vi "Describe Comparison.vi"(6 "Delta":variant, 7 "Style":enum16{"Diff", "Plain"}(ring), 9 "Actual":variant, 10 "Expected":variant) -> (2 "Description":string)   [LabVIEW 2020, in "Utilities.lvlib"]
uses:
  Utilities.lvlib
  <vilib>/Utility/Data Type/NI_Data Type.lvlib
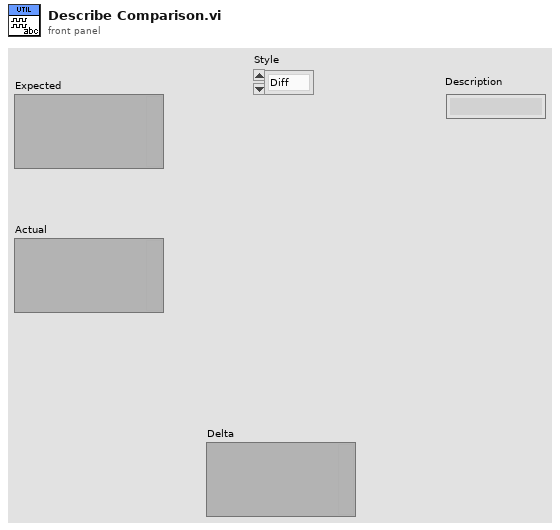
[diagram p1: front panel]
types:
  T1 = typedef "NI_Data Type.lvlib/Data Type.ctl" = enum8{"Invalid Type", "Void", "I8", "I16", "I32", "I64", "U8", "U16", "U32", "U64", "Single Float", "Double Float", "Extended Float", "Single Complex", "Double Complex", "Extended Complex", "Enum U8", "Enum U16", "Enum U32", "Enum U64", "Single Float With Unit", "Double Float With Unit", "Extended Float With Unit", "Single Complex with Unit", "Double Complex with Unit", "Extended Complex with Unit", "Boolean", "String", "Path", "Picture", "Tag", "Array", "Cluster", "Variant", "LV Variant", "Waveform", "Timestamp", "Digital Waveform", "Digital Data", "ExpressData", "Refnum", "External Data", "VI", "Poly VI", "LabVIEW Class Instance", "Fixed Point", "Set Collection", "Map Collection"}
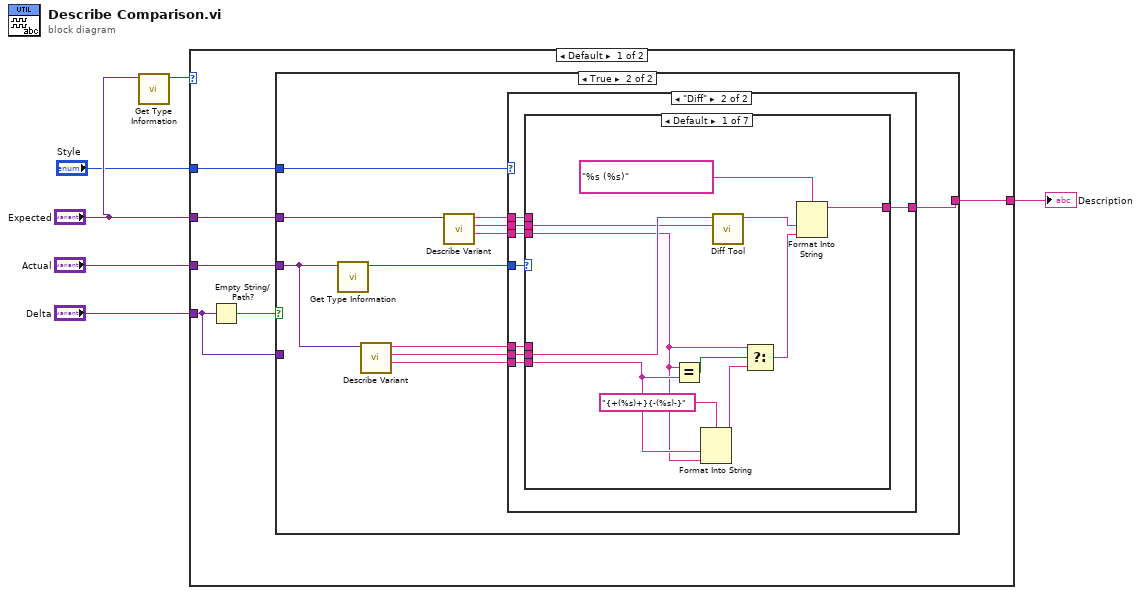
[diagram p0: block diagram]
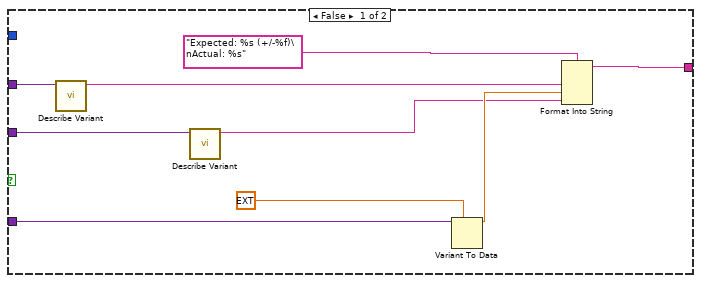
[diagram p2: hidden frame]
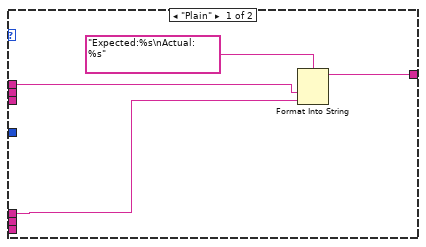
[diagram p3: hidden frame]
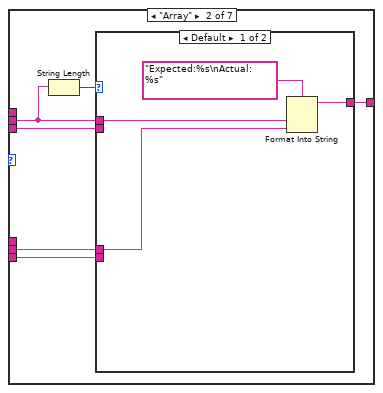
[diagram p4: hidden frame]
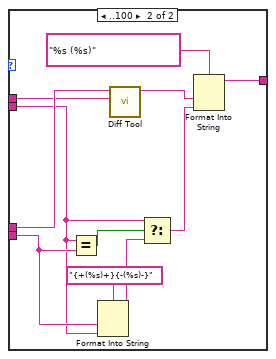
[diagram p5: hidden frame]
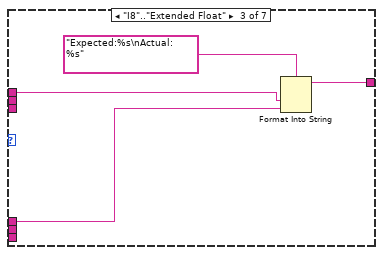
[diagram p6: hidden frame]
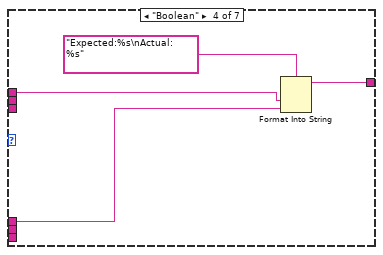
[diagram p7: hidden frame]
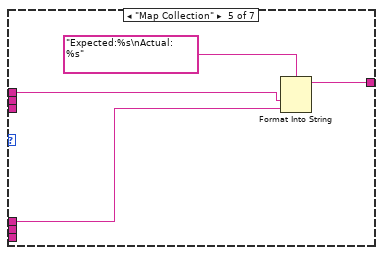
[diagram p8: hidden frame]
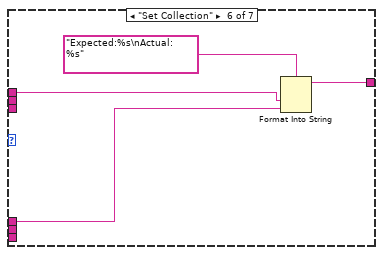
[diagram p9: hidden frame]
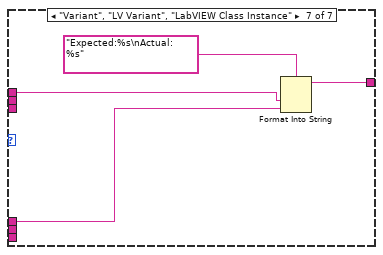
[diagram p10: hidden frame]
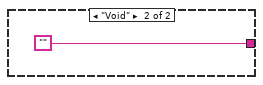
[diagram p11: hidden frame]
diagram:
  n1 = call <vilib>:"Get Type Information.vi"("variant"="Expected") -> ("type"=w2:T1)  [unwired: 6 in, 4 out]
  n2 = case shown="Default" w2 {
    tunnel: "Actual" -> [w12 _]
    tunnel: "Delta" -> [w11 _]
    tunnel: [w10 ""] -> w4
    tunnel: "Expected" -> [w8 _]
    tunnel: "Style" -> [w7 _]
    frame Default {
      n3 = Empty String/Path?(string/path=w11) -> (empty?=w9:bool)
      n4 = case shown="True" w9 {
        tunnel: w8 -> [w18 w32]
        tunnel: w12 -> [w16 w28]
        tunnel: w11 -> [w17 _]
        tunnel: [w15 w31] -> w10
        tunnel: w7 -> [_ w22]
        frame False {
          n5 = call "Describe Variant.vi"("Variant"=w18) -> ("Variant Description"=w19:string)  [unwired: 8 in, 2 out]
          n6 = call "Describe Variant.vi"("Variant"=w16) -> ("Variant Description"=w13:string)  [unwired: 8 in, 2 out]
          n7 = Variant To Data(type=ext 0.0, Variant=w17) -> (data=w14:ext)  [unwired: 1 in, 1 out]
          n8 = Format Into String(format string="Expected: %s (+/-%f)\nActual: %s", w19, w14, w13) -> (resulting string=w15:string)  [unwired: 2 in, 1 out]
        }
        frame True {
          n9 = call <vilib>:"Get Type Information.vi"("variant"=w28) -> ("type"=w27:T1)  [unwired: 6 in, 4 out]
          n10 = call "Describe Variant.vi"("Variant"=w28) -> ("Type Description"=w23:string, "Description"=w30:string, "Variant Description"=w25:string)  [unwired: 8 in]
          n11 = call "Describe Variant.vi"("Variant"=w32) -> ("Type Description"=w24:string, "Description"=w29:string, "Variant Description"=w26:string)  [unwired: 8 in]
          n12 = case shown="\"Diff\"" w22 {
            tunnel: [w36 w44] -> w31
            tunnel: w30 -> [_ w43]
            tunnel: w29 -> [_ w42]
            tunnel: w27 -> [_ w41]
            tunnel: w26 -> [w35 w40]
            tunnel: w25 -> [w34 w39]
            tunnel: w24 -> [_ w38]
            tunnel: w23 -> [_ w37]
            frame "Plain" {
              n13 = Format Into String(format string="Expected:%s\nActual:  %s", w35, w34) -> (resulting string=w36:string)  [unwired: 2 in, 1 out]
            }
            frame "Diff" {
              n14 = case shown="Default" w41 {
                tunnel: [w55 w61 w79 w83 w87 w91 w95] -> w44
                tunnel: w43 -> [w54 w60 _ _ _ _ _]
                tunnel: w42 -> [w53 w57 _ _ _ _ _]
                tunnel: w40 -> [_ _ w78 w82 w86 w90 w94]
                tunnel: w39 -> [_ _ w77 w81 w85 w89 w93]
                tunnel: w38 -> [w51 w58 _ _ _ _ _]
                tunnel: w37 -> [w52 w59 _ _ _ _ _]
                frame Default {
                  n15 = Equal?(x=w51, y=w52) -> (x = y?=w48:bool)
                  n16 = Format Into String(format string="{+(%s)+}{-(%s)-}", w52, w51) -> (resulting string=w45:string)  [unwired: 2 in, 1 out]
                  n17 = call "Diff Tool.vi"("Reference"=w53, "Target"=w54) -> ("Result"=w49:string)  [unwired: 8 in, 1 out]
                  n18 = Select(t=w51, s=w48, f=w45) -> (s? t:f=w47:string)
                  n19 = Format Into String(format string="%s (%s)", w49, w47) -> (resulting string=w55:string)  [unwired: 2 in, 1 out]
                }
                frame "Array" {
                  n20 = String Length(string=w57) -> (length=w56:i32)
                  n21 = case shown="Default" w56 {
                    tunnel: [w62 w76] -> w61
                    tunnel: w60 -> [w63 w75]
                    tunnel: w59 -> [_ w74]
                    tunnel: w58 -> [_ w73]
                    tunnel: w57 -> [w64 w66]
                    frame Default {
                      n22 = Format Into String(format string="Expected:%s\nActual:  %s", w64, w63) -> (resulting string=w62:string)  [unwired: 2 in, 1 out]
                    }
                    frame ..100 {
                      n23 = Equal?(x=w73, y=w74) -> (x = y?=w70:bool)
                      n24 = Format Into String(format string="{+(%s)+}{-(%s)-}", w74, w73) -> (resulting string=w67:string)  [unwired: 2 in, 1 out]
                      n25 = call "Diff Tool.vi"("Reference"=w66, "Target"=w75) -> ("Result"=w71:string)  [unwired: 8 in, 1 out]
                      n26 = Select(t=w73, s=w70, f=w67) -> (s? t:f=w69:string)
                      n27 = Format Into String(format string="%s (%s)", w71, w69) -> (resulting string=w76:string)  [unwired: 2 in, 1 out]
                    }
                  }
                }
                frame "I8".."Extended Float" {
                  n28 = Format Into String(format string="Expected:%s\nActual:  %s", w78, w77) -> (resulting string=w79:string)  [unwired: 2 in, 1 out]
                }
                frame "Boolean" {
                  n29 = Format Into String(format string="Expected:%s\nActual:  %s", w82, w81) -> (resulting string=w83:string)  [unwired: 2 in, 1 out]
                }
                frame "Map Collection" {
                  n30 = Format Into String(format string="Expected:%s\nActual:  %s", w86, w85) -> (resulting string=w87:string)  [unwired: 2 in, 1 out]
                }
                frame "Set Collection" {
                  n31 = Format Into String(format string="Expected:%s\nActual:  %s", w90, w89) -> (resulting string=w91:string)  [unwired: 2 in, 1 out]
                }
                frame "Variant", "LV Variant", "LabVIEW Class Instance" {
                  n32 = Format Into String(format string="Expected:%s\nActual:  %s", w94, w93) -> (resulting string=w95:string)  [unwired: 2 in, 1 out]
                }
              }
            }
          }
        }
      }
    }
    frame "Void" {
    }
  }
  "Description" <- w4
